vi "Read Virtual Folder.vi"(11 "Test Runner.Project in":refnum<class "Test Runner.Project.lvclass">) -> (2 "Virtual Folder":string, 3 "Test Runner.Project out":refnum<class "Test Runner.Project.lvclass">)   [LabVIEW 2013, in "Caraya.lvlib" / "Test Runner.Project.lvclass"]
uses:
  Test Runner.Project.lvclass
  Test Runner.Project.lvclass/Test Runner.Project.ctl
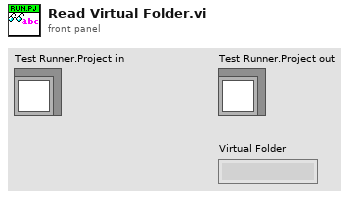
[diagram p1: front panel]
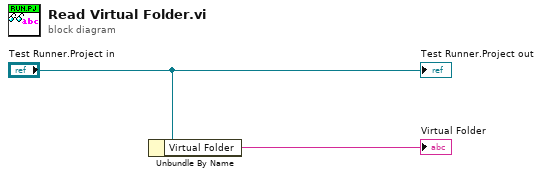
[diagram p0: block diagram]
diagram:
  n1 = Unbundle By Name("Test Runner.Project in") -> ("Virtual Folder"=→"Virtual Folder":string)
  "Test Runner.Project out" <- "Test Runner.Project in"
